vi "Create Message Accessor.vi"(8 "error in (no error)":errorcluster, 10 "Message Name":string, 11 "Library":refnum<vi>) -> (0 "error out":errorcluster, 3 "Library":refnum<vi>)   [LabVIEW 2019, in "gRPC Template Creation Utility.lvlib"]
uses:
  gRPC Template Creation Utility.lvlib
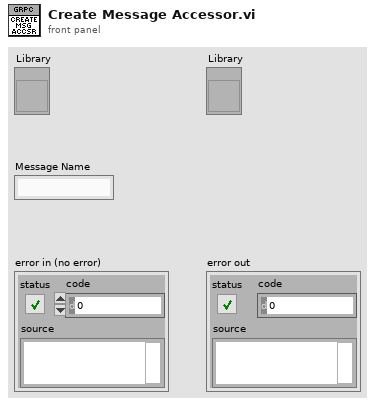
[diagram p1: front panel]
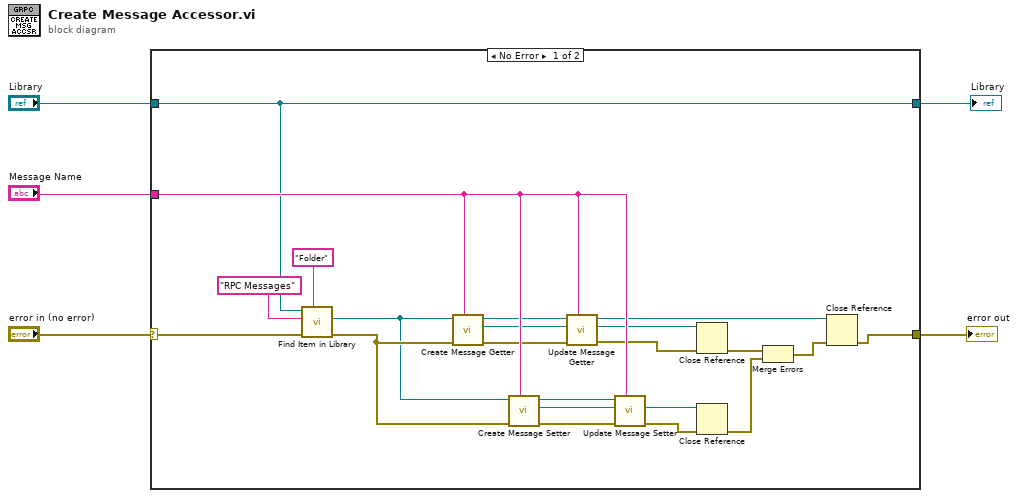
[diagram p0: block diagram]
diagram:
  n1 = case shown="No Error" "error in (no error)" {
    selector: "error in (no error)" -> [w7 w28]
    tunnel: "Library" -> [w6 w29]
    tunnel: "Message Name" -> [w27 _]
    tunnel: [w8 w28] -> w4
    tunnel: [w6 w29] -> w2
    frame No Error {
      n2 = call "Find Item in Library.vi"("Item Type"="Folder", "error in (no error)"=w7, "Item Name"="RPC Messages", "Library item in"=w6) -> ("error out"=w19:errorcluster, "Project Item (Library Item)"=w18:refnum<vi>)  [unwired: 4 in, 2 out]
      n3 = call "Create Message Getter.vi"("RPC Message Name"=w27, "error in (no error)"=w19, "RPC Messages Folder (ProjectItem) in"=w18) -> ("error out"=w22:errorcluster, "Message Getter out"=w23:refnum<vi>, "RPC Messages Folder (ProjectItem) out"=w24:refnum<vi>)  [unwired: 6 in]
      n4 = call "Create Message Setter.vi"("RPC Message Name"=w27, "error in (no error)"=w19, "RPC Messages Folder (ProjectItem) in"=w18) -> ("error out"=w17:errorcluster, "Message Setter out"=w15:refnum<vi>, "RPC Messages Folder (ProjectItem) out"=w16:refnum<vi>)  [unwired: 6 in]
      n5 = call "Update Message Getter.vi"("RPC Message Name"=w27, "error in (no error)"=w22, "Message Getter in"=w23, "RPC Messages Folder (ProjectItem) in"=w24) -> ("error out"=w20:errorcluster, "Message Getter out"=w21:refnum<vi>, "RPC Messages Folder (ProjectItem) out"=w10:refnum<vi>)  [unwired: 5 in]
      n6 = call "Update Message Setter.vi"("RPC Message Name"=w27, "error in (no error)"=w17, "Message Getter in"=w15, "RPC Messages Folder (ProjectItem) in"=w16) -> ("error out"=w14:errorcluster, "Message Getter out"=w11:refnum<vi>)  [unwired: 5 in, 1 out]
      n7 = Close Reference(reference=w21, error in (no error)=w20) -> (error out=w13:errorcluster)
      n8 = Close Reference(reference=w11, error in (no error)=w14) -> (error out=w12:errorcluster)
      n9 = Merge Errors(w13, w12) -> (w9:errorcluster)
      n10 = Close Reference(reference=w10, error in (no error)=w9) -> (error out=w8:errorcluster)
    }
    frame Error {
    }
  }
  "error out" <- w4
  "Library" <- w2
